vi "Prop Valve Set Value MW100.vi"(8 "error in (no error)":errorcluster, 10 "AO Data":dbl[](array[numeric]), 11 "MW100 Data Cluster":T1) -> (0 "error out":errorcluster, 3 "output cluster":T1)   [LabVIEW 2020]
uses:
  Type Definitions/HEWH MW100 Data Cluster.ctl
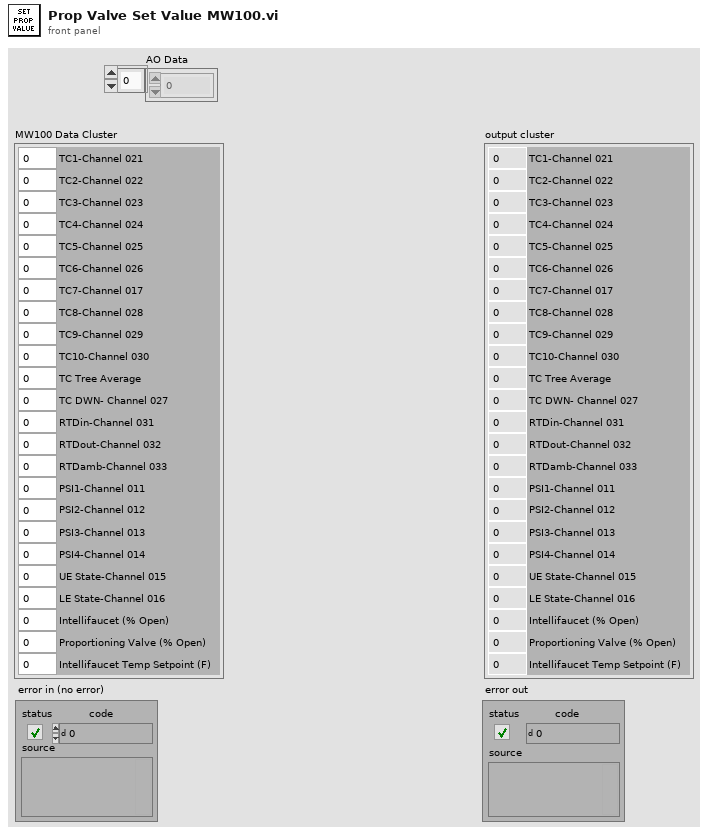
[diagram p1: front panel]
types:
  T1 = typedef "HEWH MW100 Data Cluster.ctl" = cluster{"TC1-Channel 021":dbl, "TC2-Channel 022":dbl, "TC3-Channel 023":dbl, "TC4-Channel 024":dbl, "TC5-Channel 025":dbl, "TC6-Channel 026":dbl, "TC7-Channel 017":dbl, "TC8-Channel 028":dbl, "TC9-Channel 029":dbl, "TC10-Channel 030":dbl, "TC Tree Average":dbl, "TC DWN- Channel 027":dbl, "RTDin-Channel 031":dbl, "RTDout-Channel 032":dbl, "RTDamb-Channel 033":dbl, "PSI1-Channel 011":dbl, "PSI2-Channel 012":dbl, "PSI3-Channel 013":dbl, "PSI4-Channel 014":dbl, "UE State-Channel 015":dbl, "LE State-Channel 016":dbl, "Intellifaucet (% Open)":dbl, "Proportioning Valve (% Open)":dbl, "Intellifaucet Temp Setpoint (F)":dbl}
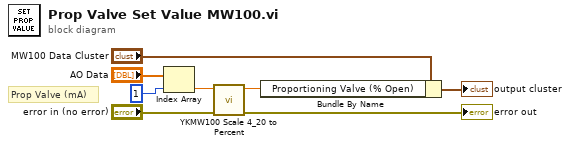
[diagram p0: block diagram]
diagram:
  # "Prop Valve (mA)"
  n1 = Index Array(array="AO Data", index=1) -> (element=w1:dbl)
  n2 = call "YKMW100 Scale 4_20 to Percent.vi"("error in (no error)"="error in (no error)", "mA"=w1) -> ("error out"=→"error out":errorcluster, "Valve (% Open)"=w8:dbl)  [unwired: 8 in]
  n3 = Bundle By Name(cluster="MW100 Data Cluster", "Proportioning Valve (% Open)"=w8) -> (→"output cluster":T1)
